vi "Diagnostics.vi"() -> ()   [LabVIEW 2015, in "Modbus Library.lvlib" / "Modbus Master.lvclass"]
uses:
  Modbus Master.lvclass
  Master Function Definition/Diagnostics Subfuntion Options.ctl
  Modbus Master.lvclass/Modbus Master.ctl
  Modbus API.lvclass/Modbus API.ctl
  Transmission Data Unit/Transmission Data Unit.lvclass
  Modbus API.lvclass
  Master Function Definition/Master Function Definition.lvclass
panel:
  out "Data":u16[](array[numeric])
  in  "Data":u16[](array[numeric])
  in  "Sub-function":T1 items=["Return Query Data"=0, "Restart Communications Option"=1, "Return Diagnostic Register"=2, "Change ASCII Input Delimiter"=3, "Force Listen Only Mode"=4, "Clear Counters and Diagnostic Register"=10, "Return Bus Message Count"=11, "Return Bus Communication Error Count"=12, "Return Bus Exception Error Count"=13, "Return Slave Message Count"=14, "Return Slave No Response Count"=15, "Return Slave NAK Count"=16, "Return Slave Busy Count"=17, "Return Bus Character Overrun Count"=18, "Clear Overrun Counter and Flag"=20]
  out "Modbus master out":refnum<class "Modbus Master.lvclass">
  in  "Modbus master in":refnum<class "Modbus Master.lvclass">
  out "error out":errorcluster
  in  "error in":errorcluster
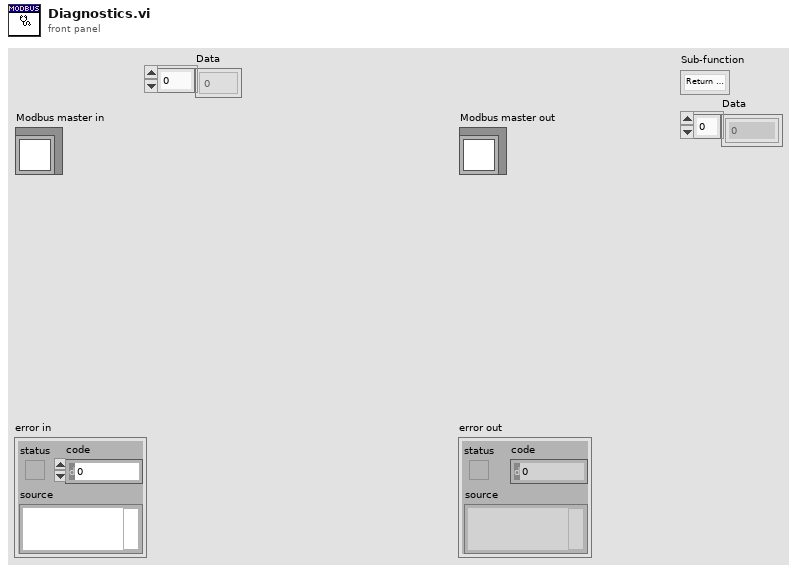
[diagram p1: front panel]
types:
  T1 = typedef "Diagnostics Subfuntion Options.ctl" = u16
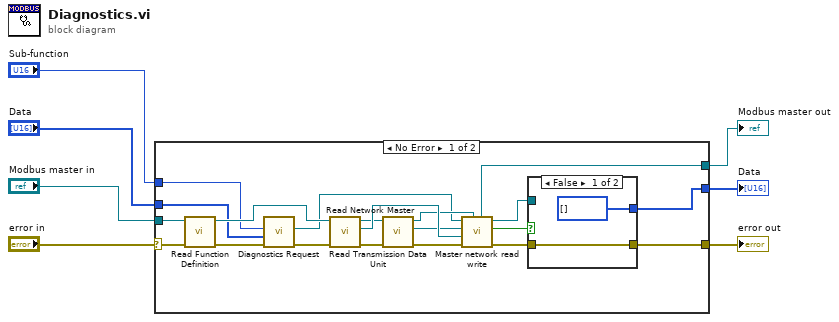
[diagram p0: block diagram]
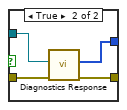
[diagram p2: hidden frame]
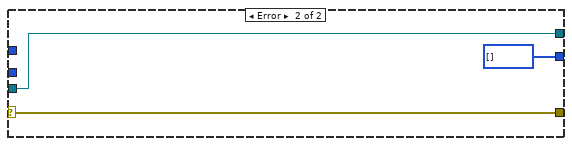
[diagram p3: hidden frame]
diagram:
  n1 = case shown="No Error" "error in" {
    selector: "error in" -> [w24 w36]
    tunnel: [w23 w36] -> w5
    tunnel: [w20 w35] -> w6
    tunnel: "Modbus master in" -> [w25 w35]
    tunnel: "Sub-function" -> [w11 _]
    tunnel: "Data" -> [w10 _]
    tunnel: [w8 u16[] [] ("Data")] -> w1
    frame No Error {
      n2 = call "Read Function Definition.vi"("error in"=w24, "Modbus master in"=w25) -> ("error out"=w13:errorcluster, "Modbus master out"=w16:refnum<class "Modbus Master.lvclass">)  [unwired: 7 in, 1 out]
      n3 = call "Diagnostics Request.vi"("error in (no error)"=w13, "Data"=w10, "Sub-function"=w11) -> ("error out"=w12:errorcluster, "modbus data unit out"=w9:refnum<class "Modbus Data Unit.lvclass">)  [unwired: 7 in]
      n4 = call "Read Transmission Data Unit.vi"("error in"=w12, "Modbus instance in"=w16) -> ("error out"=w18:errorcluster, "transmission data unit"=w22:refnum<class "Transmission Data Unit.lvclass">, "Modbus instance out"=w17:refnum<class "Modbus Master.lvclass">)  [unwired: 7 in]
      n5 = call "Read Network Master.vi"("error in"=w18, "Modbus master in"=w17) -> ("error out"=w19:errorcluster, "network master"=w21:refnum<class "Network Master.lvclass">, "Modbus master out"=w15:refnum<class "Modbus Master.lvclass">)  [unwired: 7 in]
      n6 = call "Master network read write.vi"("Modbus master in"=w15, "error in"=w19, "transmission data unit in"=w22, "network master in"=w21, "Modbus data unit in"=w9) -> ("error out"=w26:errorcluster, "PDU Valid?"=w14:bool, "Modbus data unit out"=w27:refnum<class "Modbus Data Unit.lvclass">, "Modbus master out"=w20:refnum<class "Modbus Master.lvclass">)  [unwired: 3 in]
      n7 = case shown="False" w14 {
        tunnel: w27 -> [_ w33]
        tunnel: w26 -> [w29 w32]
        tunnel: [w29 w31] -> w23
        tunnel: [u16[] [] ("Data") w30] -> w8
        frame False {
        }
        frame True {
          n8 = call "Diagnostics Response.vi"("error in (no error)"=w32, "Modbus Library.lvlib:Modbus Data Unit"=w33) -> ("error out"=w31:errorcluster, "Data"=w30:u16[])  [unwired: 8 in]
        }
      }
    }
    frame Error {
    }
  }
  "error out" <- w5
  "Modbus master out" <- w6
  "Data" <- w1
